vi "Assert Error.vi"(8 "Error":errorcluster, 10 "Error String":string) -> (2 "Success":bool)   [LabVIEW 2024]
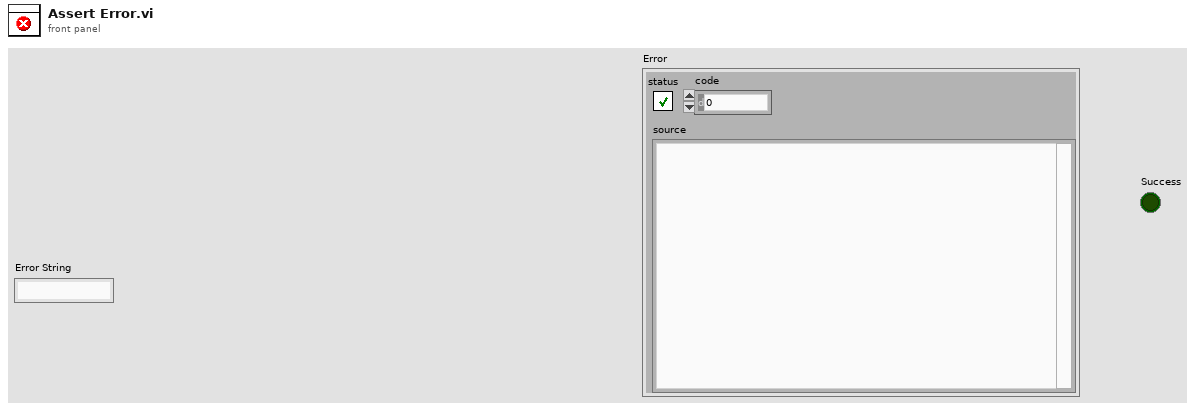
[diagram p1: front panel]
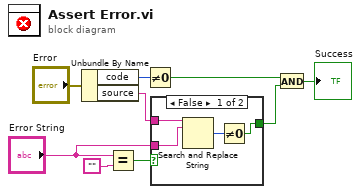
[diagram p0: block diagram]
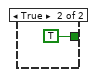
[diagram p2: hidden frame]
diagram:
  n1 = Unbundle By Name("Error") -> ("code"=w9:i32, "source"=w3:string)
  n2 = Equal?(x="Error String", y="") -> (x = y?=w6:bool)
  n3 = Not Equal To 0?(x=w9) -> (x != 0?=w2:bool)
  n4 = case shown="False" w6 {
    tunnel: [w10 TRUE] -> w5
    tunnel: "Error String" -> [w13 _]
    tunnel: w3 -> [w12 _]
    frame False {
      n5 = Search and Replace String(input string=w12, search string=w13) -> (number of replacements=w11:i32)  [unwired: 6 in, 3 out]
      n6 = Not Equal To 0?(x=w11) -> (x != 0?=w10:bool)
    }
    frame True {
    }
  }
  n7 = And(x=w2, y=w5) -> (x .and. y?=→"Success":bool)
